vi "add_configuration_item.vi"(8 "error in (no error)":errorcluster) -> (0 "error out":errorcluster, 2 "canceled?":bool, 3 "additional-component config name 2":string)   [LabVIEW 2010]
panel:
  in  "button: cancel":bool
  in  "button: add configuration":bool
  in  "additional-component config name":string caption="configuration name"
  # "Create configuration for listed component"
  # "Select a component above and enter a new configuration name here."
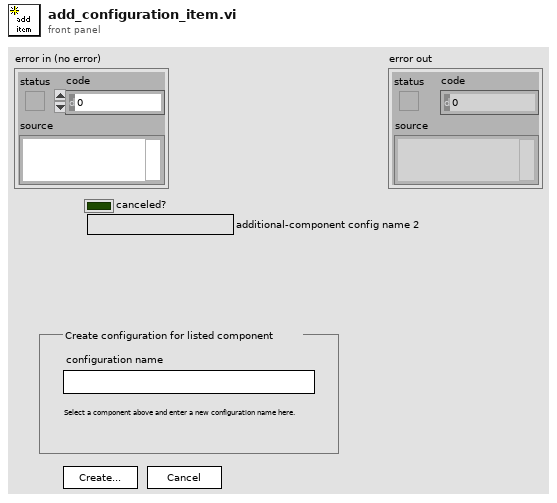
[diagram p1: front panel]
types:
  T1 = enum8{"Enabled", "Disabled", "Disabled and Grayed Out"}
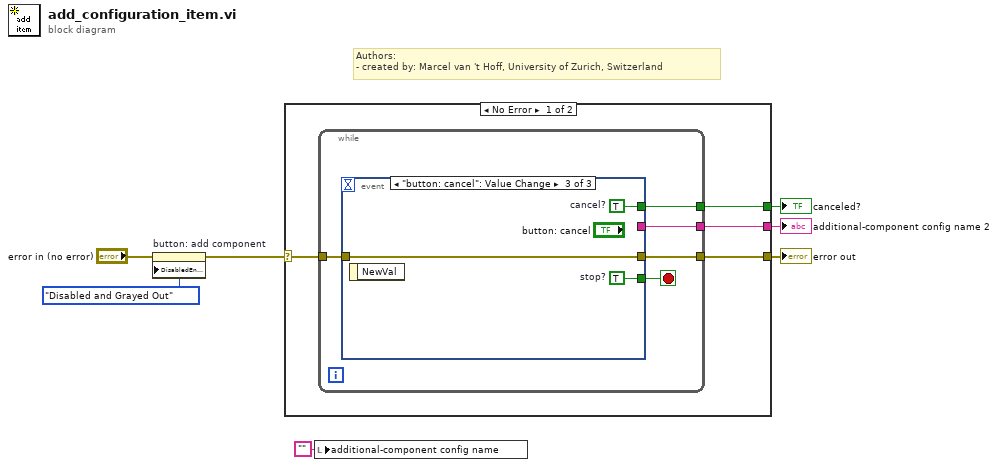
[diagram p0: block diagram]
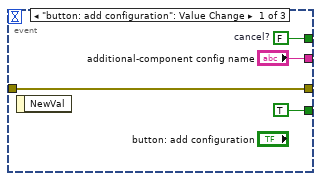
[diagram p2: hidden frame]
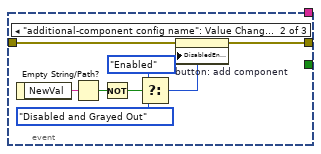
[diagram p3: hidden frame]
diagram:
  # "Authors: \n- created by: Marcel van 't Hoff, University of Zurich, Switzerland"
  n1 = property on="button: add component" class="Bool"(error in="error in (no error)", "DisabledEnum"=T1."Disabled and Grayed Out" ("Disabled")) -> (error out=w2:errorcluster)  [unwired: 1 in, 1 out]
  n2 = case shown="No Error" w2 {
    selector: w2 -> [w10 w32]
    tunnel: [w11 w32] -> w7
    tunnel: [w9 _] -> w6
    tunnel: [w8 _] -> w4
    frame No Error {
      n3 = while {
        tunnel: [w16] -> w11
        tunnel: w10 -> [w15]
        tunnel: [w14] -> w9
        tunnel: [w12] -> w8
        stop <- w13 stop-if-true
        n4 = event shown="[2] \"button: cancel\": Value Change" {
          selector: _ -> [_ _ _]
          dyn-events: _ -> [_ _ _]
          timeout: _ -> [_ _ _]
          tunnel: [w20 w26 w31] -> w16
          tunnel: w15 -> [w20 w27 w31]
          tunnel: ["additional-component config name" _ _] -> w14
          tunnel: [TRUE ("stop?") _ w30] -> w13
          tunnel: [w18 _ w29] -> w12
          event "button: add configuration": Value Change {
            w18 = FALSE  # cancel?
            n5 = event-data() -> ()  [unwired: 1 in, 1 out]
          }
          event "additional-component config name": Value Change {
            n6 = event-data() -> ("NewVal"=w21:string)  [unwired: 1 in]
            n7 = Empty String/Path?(string/path=w21) -> (empty?=w28:bool)
            n8 = Not(x=w28) -> (.not. x?=w24:bool)
            n9 = Select(t=T1."Enabled" ("Disabled"), s=w24, f=T1."Disabled and Grayed Out") -> (s? t:f=w23:T1)
            n10 = property on="button: add component" class="Bool"(error in=w27, "DisabledEnum"=w23) -> (error out=w26:errorcluster)  [unwired: 1 in, 1 out]
          }
          event "button: cancel": Value Change {
            w29 = TRUE  # cancel?
            w30 = TRUE  # stop?
            n11 = event-data() -> ()  [unwired: 1 in, 1 out]
          }
        }
      }
    }
    frame Error {
    }
  }
  "error out" <- w7
  "additional-component config name 2" <- w6
  "canceled?" <- w4
  n12 = local write "additional-component config name"("") -> ()
